vi "Get Metadata.vi"(8 "error in (no error)":errorcluster, 10 "stream index":i32, 11 "refnum in":refnum<k20>) -> (0 "error out":errorcluster, 2 "elements per cycle":u8, 3 "refnum out":refnum<k20>)   [LabVIEW 2015, in "niInstr Streaming v1 Host.lvlib"]
doc: "This is an internal interface, but is made public access to facilitate extension. The metadata that the stream reports will be accessibled via this interface.\n\n<B>Input Parameters</B>\n\n<B>error in (no error)</B> 'error in' can accept error information wired from VIs previously called. Use this information to decide if any functionality should be bypassed in the event of errors from other VIs.\n\nRight-click the 'error in' control on the front panel and select 'Explain Error' or 'Explain Warning' from the shortcut menu for more information about the error.\n\n<B>stream index</B> Selects which stream index this VI will interface to. This is the index number at the end of the host interface controls (0..7).\n\n<B>refnum in</B> Wire in the session obtained from Open FPGA Reference.\n\n<B>Output Parameters</B>\n\n<B>error out</B> contains error information. This output provides standard error out functionality.\n\n<B>refnum out</B> Copy of refnum in"
uses:
  <instrlib>/_niInstr/Streaming/v1/Host/niInstr Streaming v1 Host.lvlib
  <instrlib>/_niInstr/Streaming/v1/Host/Public/Stream Host Interface.ctl
  <vilib>/Utility/error.llb/Error Cluster From Error Code.vi
  <vilib>/rvi/errors/niLvFpgaAdjustHostInterfaceError.vi
  <vilib>/ErrorRing/Error Ring.xnode
  <vilib>/rvi/interface/nirviReadWriteControl/nirviReadWriteControl.xnode
  <vilib>/rvi/interface/Simulation/niFpgaSimulationCallBeginRW.vi
  NiFpgaLv.dll
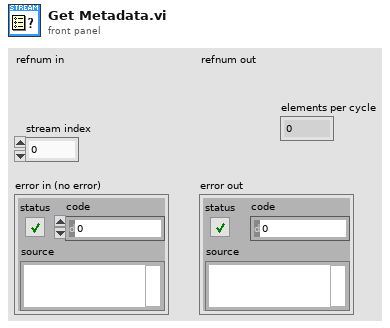
[diagram p1: front panel]
types:
  T1 = typedef "niInstr Streaming v1 Host.lvlib/Stream Host Interface.ctl" = refnum<k20>
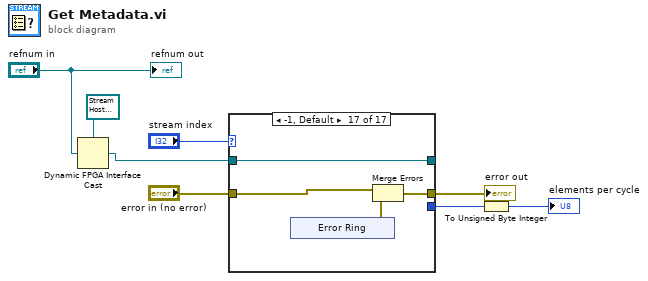
[diagram p0: block diagram]
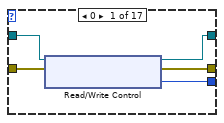
[diagram p2: hidden frame]
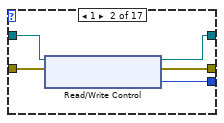
[diagram p3: hidden frame]
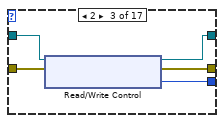
[diagram p4: hidden frame]
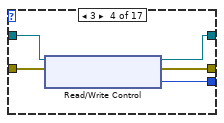
[diagram p5: hidden frame]
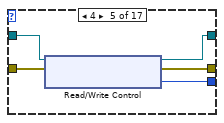
[diagram p6: hidden frame]
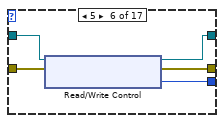
[diagram p7: hidden frame]
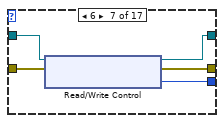
[diagram p8: hidden frame]
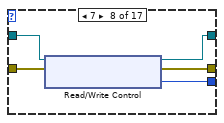
[diagram p9: hidden frame]
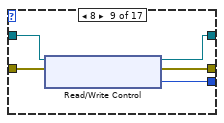
[diagram p10: hidden frame]
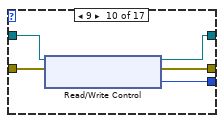
[diagram p11: hidden frame]
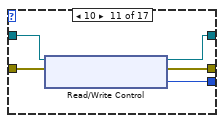
[diagram p12: hidden frame]
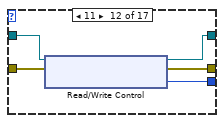
[diagram p13: hidden frame]
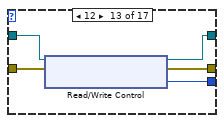
[diagram p14: hidden frame]
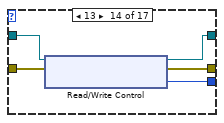
[diagram p15: hidden frame]
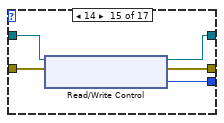
[diagram p16: hidden frame]
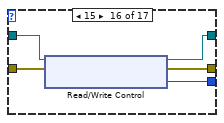
[diagram p17: hidden frame]
diagram:
  n1 = Dynamic FPGA Interface Cast(Session In=T1 refnum ("Refnum in"), Type="refnum in") -> (Session Out=w5:T1)
  n2 = case shown="-1, Default" "stream index" {
    tunnel: "error in (no error)" -> [w13 w18 w23 w28 w33 w38 w43 w48 w53 w58 w63 w68 w73 w78 w83 w88 w89]
    tunnel: [w12 w17 w22 w27 w32 w37 w42 w47 w52 w57 w62 w67 w72 w77 w82 w87 w92] -> _
    tunnel: [w11 w16 w21 w26 w31 w36 w41 w46 w51 w56 w61 w66 w71 w76 w81 w86 w90] -> w8
    tunnel: w5 -> [w10 w15 w20 w25 w30 w35 w40 w45 w50 w55 w60 w65 w70 w75 w80 w85 w92]
    tunnel: [w9 w14 w19 w24 w29 w34 w39 w44 w49 w54 w59 w64 w69 w74 w79 w84 _] -> w1
    frame 0 {
      n3 = xnode ("Read/Write Control")("FPGA VI Reference In"=w10, "error in"=w13) -> ("FPGA VI Reference Out"=w12:T1, "error out"=w11:errorcluster, "stream.metadata 0"=w9:u64)
    }
    frame 1 {
      n4 = xnode ("Read/Write Control")("FPGA VI Reference In"=w15, "error in"=w18) -> ("FPGA VI Reference Out"=w17:T1, "error out"=w16:errorcluster, "stream.metadata 1"=w14:u64)
    }
    frame 2 {
      n5 = xnode ("Read/Write Control")("FPGA VI Reference In"=w20, "error in"=w23) -> ("FPGA VI Reference Out"=w22:T1, "error out"=w21:errorcluster, "stream.metadata 2"=w19:u64)
    }
    frame 3 {
      n6 = xnode ("Read/Write Control")("FPGA VI Reference In"=w25, "error in"=w28) -> ("FPGA VI Reference Out"=w27:T1, "error out"=w26:errorcluster, "stream.metadata 3"=w24:u64)
    }
    frame 4 {
      n7 = xnode ("Read/Write Control")("FPGA VI Reference In"=w30, "error in"=w33) -> ("FPGA VI Reference Out"=w32:T1, "error out"=w31:errorcluster, "stream.metadata 4"=w29:u64)
    }
    frame 5 {
      n8 = xnode ("Read/Write Control")("FPGA VI Reference In"=w35, "error in"=w38) -> ("FPGA VI Reference Out"=w37:T1, "error out"=w36:errorcluster, "stream.metadata 5"=w34:u64)
    }
    frame 6 {
      n9 = xnode ("Read/Write Control")("FPGA VI Reference In"=w40, "error in"=w43) -> ("FPGA VI Reference Out"=w42:T1, "error out"=w41:errorcluster, "stream.metadata 6"=w39:u64)
    }
    frame 7 {
      n10 = xnode ("Read/Write Control")("FPGA VI Reference In"=w45, "error in"=w48) -> ("FPGA VI Reference Out"=w47:T1, "error out"=w46:errorcluster, "stream.metadata 7"=w44:u64)
    }
    frame 8 {
      n11 = xnode ("Read/Write Control")("FPGA VI Reference In"=w50, "error in"=w53) -> ("FPGA VI Reference Out"=w52:T1, "error out"=w51:errorcluster, "stream.metadata 8"=w49:u64)
    }
    frame 9 {
      n12 = xnode ("Read/Write Control")("FPGA VI Reference In"=w55, "error in"=w58) -> ("FPGA VI Reference Out"=w57:T1, "error out"=w56:errorcluster, "stream.metadata 9"=w54:u64)
    }
    frame 10 {
      n13 = xnode ("Read/Write Control")("FPGA VI Reference In"=w60, "error in"=w63) -> ("FPGA VI Reference Out"=w62:T1, "error out"=w61:errorcluster, "stream.metadata 10"=w59:u64)
    }
    frame 11 {
      n14 = xnode ("Read/Write Control")("FPGA VI Reference In"=w65, "error in"=w68) -> ("FPGA VI Reference Out"=w67:T1, "error out"=w66:errorcluster, "stream.metadata 11"=w64:u64)
    }
    frame 12 {
      n15 = xnode ("Read/Write Control")("FPGA VI Reference In"=w70, "error in"=w73) -> ("FPGA VI Reference Out"=w72:T1, "error out"=w71:errorcluster, "stream.metadata 12"=w69:u64)
    }
    frame 13 {
      n16 = xnode ("Read/Write Control")("FPGA VI Reference In"=w75, "error in"=w78) -> ("FPGA VI Reference Out"=w77:T1, "error out"=w76:errorcluster, "stream.metadata 13"=w74:u64)
    }
    frame 14 {
      n17 = xnode ("Read/Write Control")("FPGA VI Reference In"=w80, "error in"=w83) -> ("FPGA VI Reference Out"=w82:T1, "error out"=w81:errorcluster, "stream.metadata 14"=w79:u64)
    }
    frame 15 {
      n18 = xnode ("Read/Write Control")("FPGA VI Reference In"=w85, "error in"=w88) -> ("FPGA VI Reference Out"=w87:T1, "error out"=w86:errorcluster, "stream.metadata 15"=w84:u64)
    }
    frame -1, Default {
      n19 = xnode "Error Ring"() -> ("error out"=w91:errorcluster)
      n20 = Merge Errors(w89, w91) -> (w90:errorcluster)
    }
  }
  "error out" <- w8
  n21 = To Unsigned Byte Integer(number=w1) -> (unsigned 8bit integer=→"elements per cycle":u8)
  "refnum out" <- "refnum in"
